vi "Edit-dialog.vi"(8 "error in (no error)":errorcluster, 11 "Action in":refnum<class "Move-Absolute.lvclass">) -> (0 "error out":errorcluster, 3 "Action out":refnum<class "Move-Absolute.lvclass">)   [LabVIEW 2013, in "PowderDeposition.lvlib" / "Move-Absolute.lvclass"]
uses:
  Move-Absolute.lvclass
  Move-Absolute-settings.ctl
  Move-Absolute.lvclass/Move-Absolute.ctl
panel:
  in  "Cancel":bool
  in  "OK":bool
  in  "Edit dialog":T1
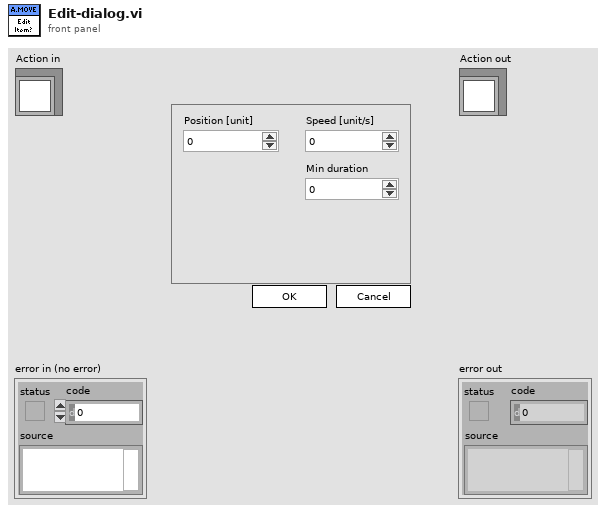
[diagram p1: front panel]
types:
  T1 = typedef "PowderDeposition.lvlib/Move-Absolute.lvclass/Move-Absolute-settings.ctl" = cluster{"Position":dbl, "Speed":dbl, "Min duration":dbl}
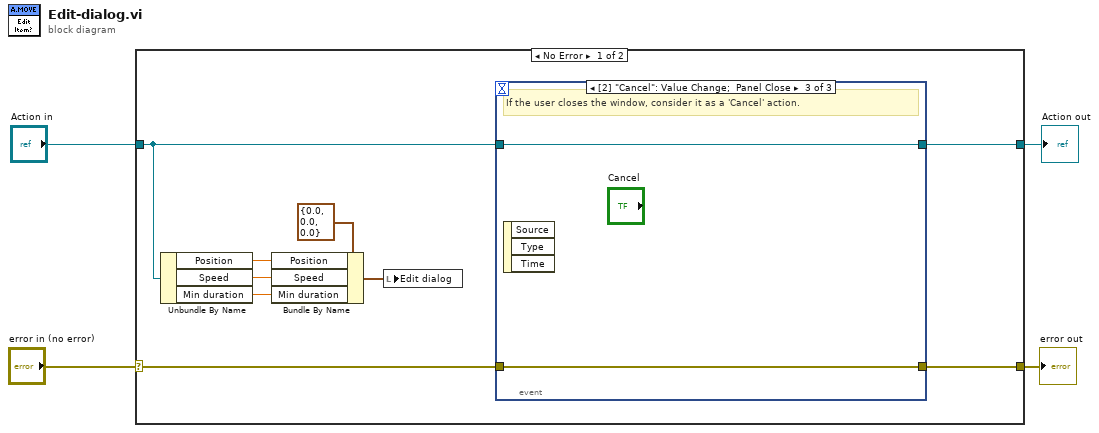
[diagram p0: block diagram]
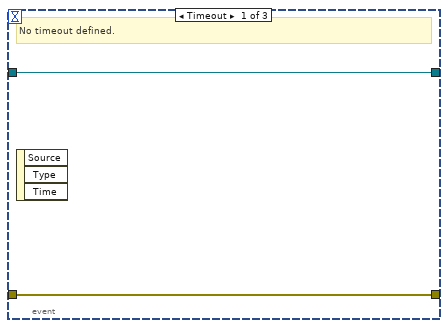
[diagram p2: hidden frame]
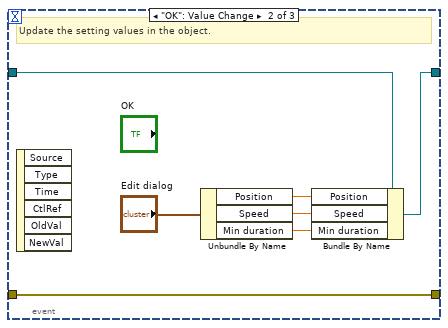
[diagram p3: hidden frame]
diagram:
  n1 = case shown="No Error" "error in (no error)" {
    selector: "error in (no error)" -> [w12 w26]
    tunnel: [w11 w26] -> w3
    tunnel: [w13 w25] -> w1
    tunnel: "Action in" -> [w6 w25]
    frame No Error {
      n2 = Unbundle By Name(w6) -> ("Position"=w7:dbl, "Speed"=w8:dbl, "Min duration"=w9:dbl)
      n3 = Bundle By Name(cluster=T1 {"Position"=0.0, "Speed"=0.0, "Min duration"=0.0} ("Edit dialog"), "Position"=w7, "Speed"=w8, "Min duration"=w9) -> (w10:T1)
      n4 = local write "Edit dialog"(w10) -> ()
      n5 = event shown="[2] \"Cancel\": Value Change;  Panel Close" {
        selector: _ -> [_ _ _]
        dyn-events: _ -> [_ _ _]
        timeout: _ -> [_ _ _]
        tunnel: w6 -> [w15 w21 w24]
        tunnel: [w15 w20 w24] -> w13
        tunnel: w12 -> [w14 w22 w23]
        tunnel: [w14 w22 w23] -> w11
        event Timeout {
          # "No timeout defined."
          n6 = event-data() -> ()  [unwired: 1 in, 3 out]
        }
        event "OK": Value Change {
          # "Update the setting values in the object."
          n7 = event-data() -> ()  [unwired: 1 in, 6 out]
          n8 = Unbundle By Name("Edit dialog") -> ("Position"=w18:dbl, "Speed"=w17:dbl, "Min duration"=w16:dbl)
          n9 = Bundle By Name(cluster=w21, "Position"=w18, "Speed"=w17, "Min duration"=w16) -> (w20:refnum<class "Move-Absolute.lvclass">)
        }
        event "Cancel": Value Change; Panel Close {
          # "If the user closes the window, consider it as a 'Cancel' action."
          n10 = event-data() -> ()  [unwired: 1 in, 3 out]
        }
      }
    }
    frame Error {
    }
  }
  "error out" <- w3
  "Action out" <- w1
